vi "ILM_Split_Cluster.vi"(0 "SR830-2 2":T3 {"Nitrogen" format="%#4_5f"}) -> (1 "SR830-2 4":T1 {"Nitrogen" format="%#4_5f"}, 2 "SR830-2 3":T2)   [LabVIEW 2018]
uses:
  S16/ILM-Cluster.ctl
  S16/ILM-Control.ctl
  S16/ILM-Status.ctl
panel:
  # "N (%)"
  # "He (%)"
  # "Levelmeter"
  # "N (%)"
  # "He (%)"
  # "Levelmeter"
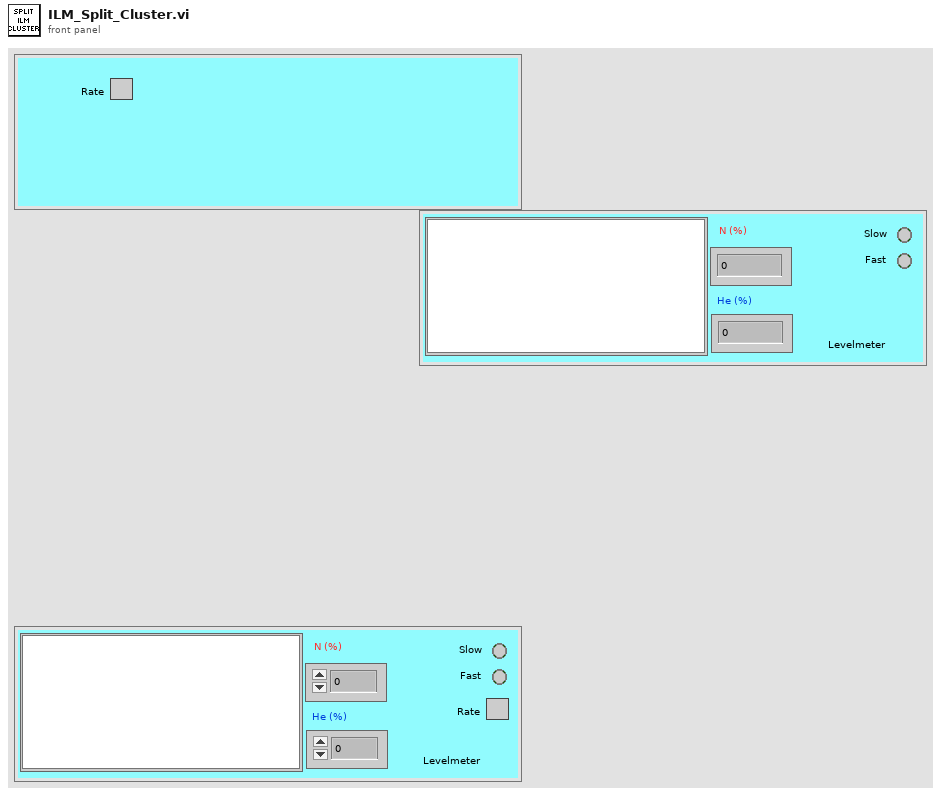
[diagram p1: front panel]
types:
  T1 = typedef "ILM-Status.ctl" = cluster{"Plot":dbl[][], "Nitrogen":dbl, "Helium":dbl, "Fast":bool, "Slow":bool}
  T2 = typedef "ILM-Control.ctl" = cluster{"Rate":bool}
  T3 = typedef "ILM-Cluster.ctl" = cluster{"Plot":dbl[][], "Nitrogen":dbl, "Helium":dbl, "Fast":bool, "Slow":bool, "Rate":bool}
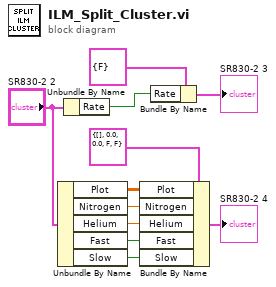
[diagram p0: block diagram]
diagram:
  n1 = Unbundle By Name("SR830-2 2") -> ("Plot"=w7:dbl[][], "Nitrogen"=w6:dbl, "Helium"=w5:dbl, "Fast"=w4:bool, "Slow"=w3:bool)
  n2 = Unbundle By Name("SR830-2 2") -> ("Rate"=w2:bool)
  n3 = Bundle By Name(cluster=T1 {"Plot"=[], "Nitrogen"=0.0, "Helium"=0.0, "Fast"=FALSE, "Slow"=FALSE} ("SR830-2 2"), "Plot"=w7, "Nitrogen"=w6, "Helium"=w5, "Fast"=w4, "Slow"=w3) -> (→"SR830-2 4":T1)
  n4 = Bundle By Name(cluster=T2 {"Rate"=FALSE} ("SR830-2 2"), "Rate"=w2) -> (→"SR830-2 3":T2)
